vi "Write PluginINIFilePath.vi"(8 "error in (no error)":errorcluster, 10 "PluginINIFilePath":path, 11 "NISTPluginsBase in":refnum<class "MyPluginsBase.lvclass">) -> (0 "error out":errorcluster, 3 "NISTPluginsBase out":refnum<class "MyPluginsBase.lvclass">)   [LabVIEW 2014]
uses:
  MyPluginsBase.lvclass
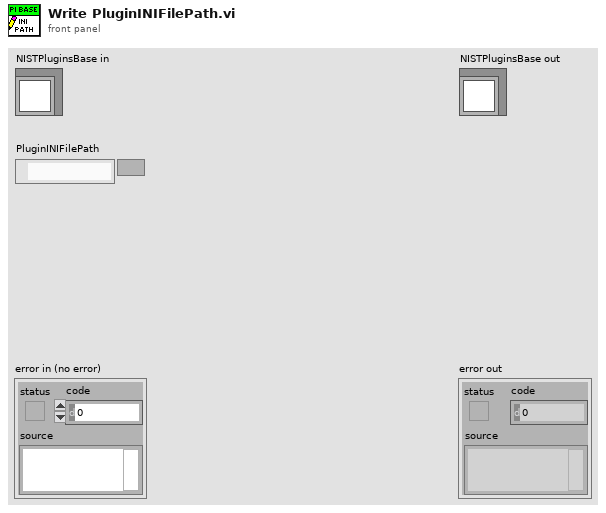
[diagram p1: front panel]
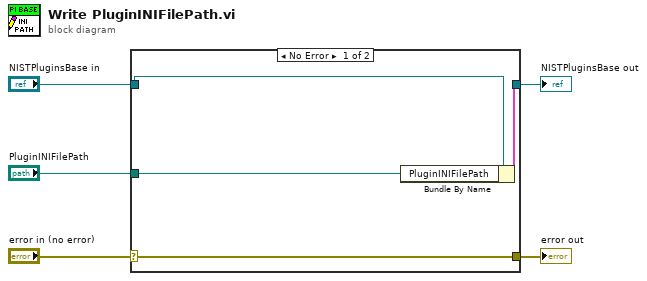
[diagram p0: block diagram]
diagram:
  n1 = case shown="No Error" "error in (no error)" {
    selector: "error in (no error)" -> [w9 w10]
    tunnel: [w9 w10] -> w4
    tunnel: [w7 w11] -> w2
    tunnel: "NISTPluginsBase in" -> [w8 w11]
    tunnel: "PluginINIFilePath" -> [w6 _]
    frame No Error {
      n2 = Bundle By Name(cluster=w8, "PluginINIFilePath"=w6) -> (w7:cluster{})
    }
    frame Error {
    }
  }
  "error out" <- w4
  "NISTPluginsBase out" <- w2
